vi "Magnetometer_Test_v1.vi"() -> ()   [LabVIEW 2019]
uses:
  <vilib>/DAQmx/write.llb/DAQmx Write (Analog DBL 1Chan 1Samp).vi
  <vilib>/DAQmx/read.llb/DAQmx Read (Analog 1D Wfm NChan NSamp).vi
  <extravilib>/ChannelInstances/Tag-bool/Write With Abort.vi
  <extravilib>/ChannelInstances/Tag-bool/Read With Abort.vi
  <extravilib>/ChannelInstances/Tag-c(bool,i32,str)/Read With Abort.vi
  <extravilib>/ChannelInstances/Tag-a[.](wfm(dbl))/Read With Abort.vi
  <extravilib>/ChannelInstances/Tag-c(bool,i32,str)/Write With Abort.vi
  <extravilib>/ChannelInstances/Tag-a[.](wfm(dbl))/Write With Abort.vi
  <vilib>/DAQmx/create/channels.llb/DAQmx Create Channel (AI-Voltage-Basic).vi
  <vilib>/DAQmx/configure/timing.llb/DAQmx Timing (Sample Clock).vi
  <vilib>/DAQmx/create/channels.llb/DAQmx Create Channel (AO-Voltage-Basic).vi
  <vilib>/Utility/file.llb/Write Delimited Spreadsheet (string).vi
  <extravilib>/ChannelInstances/Tag-a[.](wfm(dbl))/Instantiate.vi
  <extravilib>/ChannelInstances/Tag-bool/Instantiate.vi
  <extravilib>/ChannelInstances/Tag-bool/EndpointRead.vi
  <vilib>/DAQmx/miscellaneous.llb/DAQmx Fill In Error Info.vi
  <extravilib>/ChannelInstances/Tag-bool/Endpoint.vi
  <extravilib>/ChannelInstances/Tag-c(bool,i32,str)/Instantiate.vi
  <extravilib>/ChannelInstances/Tag-c(bool,i32,str)/EndpointRead.vi
  <extravilib>/ChannelInstances/Tag-a[.](wfm(dbl))/EndpointRead.vi
  <extravilib>/ChannelInstances/Tag-a[.](wfm(dbl))/Endpoint.vi
  <extravilib>/ChannelInstances/Tag-c(bool,i32,str)/Endpoint.vi
  <extravilib>/ChannelInstances/Tag-c(bool,i32,str).lvlib
  <extravilib>/ChannelInstances/Tag-a[.](wfm(dbl)).lvlib
  <extravilib>/ChannelInstances/Tag-bool.lvlib
  <resource>/objmgr/daqmx.rc
  <vilib>/DAQmx/write.llb/DAQmx Write (Analog 1D DBL NChan 1Samp).vi
panel:
  out "Temperature (VDC)":dbl
  out "Temperature":dbl(slide) scale=-40.0..160.0
  out "Magnetic Field Indicator":dbl
  out "Resistance (Ohms)":dbl
  out "Magnetic Field":dbl(graph)
  out "Temperature (Celsius)":dbl
  in  "MtM X-Axis Input Voltage":dbl
  in  "MtM Y-Axis Input Voltage":dbl
  in  "MtM Z-Axis Input Voltage":dbl
  in  "Simulation On/Off":bool
  in  "Temperature \nMeasurement On/Off":bool=TRUE
  in  "Data Record Work Rate (ms)":u16(ring)=100 items=["100"=100, "250"=250, "500"=500, "1000"=1000, "2500"=2500, "5000"=5000, ""=0]
  in  "Stop":bool
  out "Iteration of PS Controller":dbl
  out "Output 1 Measured Voltage":string
  out "Output 1 Input Voltage":string
  out "Output 1 Input Current":string
  out "Output 2 Measured Voltage":string
  out "Output 2 Measured Current":string
  out "Output 2 Input Voltage":string
  out "Output 1 Measured Current":string
  out "Output 2 Input Current":string
  in  "Reset":bool
  in  "Output On/Off":bool
  out "Output 1 Current In Range?":bool
  out "Output 2 Current In Range?":bool
  out "TCP Connection":bool
  out "MtM X-Axis Output Voltage":string
  in  "Data History Work Rate (ms)":u16(ring)=1000 items=["100"=100, "250"=250, "500"=500, "1000"=1000, "2500"=2500, "5000"=5000, ""=0]
  out "MtM Y-Axis Output Voltage":string
  out "MtM Z-Axis Output Voltage":string
  in  "Sample Clock Source":tag="OnboardClock"
  in  "Acquire Buffer Size":i32=1024
  out "While loop duration (ms)":u32
  out "DAQmx Read Rate":dbl
  in  "Number of Samples":i32=100
  out "MtM X-Axis Output Voltage 2":waveform(dbl)(graph)
  out "MtM Y-Axis Output Voltage 2":waveform(dbl)(graph)
  out "MtM Z-Axis Output Voltage 2":waveform(dbl)(graph)
  in  "Sample Rate":dbl=1000.0 format="%0.2f"
  # "Sensor Output"
  # "Data Acqusition Timing and\nBuffer Settings"
  # "Temperature Output"
  # "Acquire Data History"
  # "Magnetic Field Output"
  # "Power Supply Control and Status"
  # "Simulation of Analogue Voltage Generation"
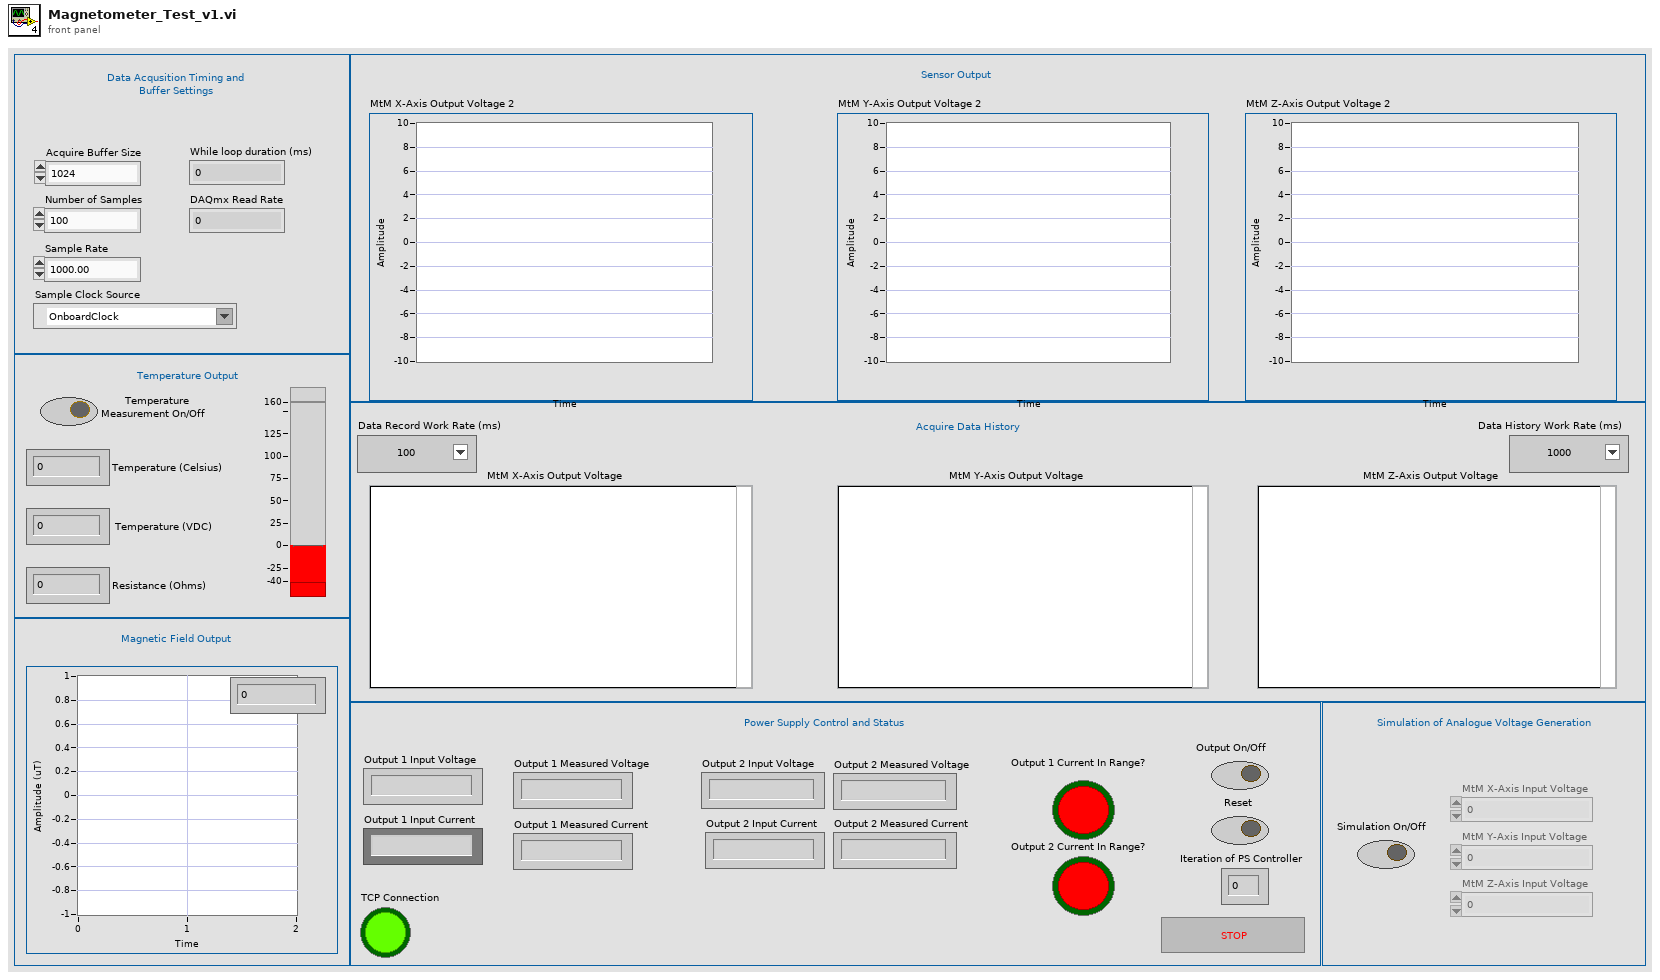
[diagram p1: front panel]
types:
  T1 = typedef "Tag-bool.lvlib/))Channel.ctl" = refnum<queue>
  T2 = enum8{"Enabled", "Disabled", "Disabled and Grayed Out"}
  T3 = typedef "Tag-a[.](wfm(dbl)).lvlib/))Channel.ctl" = refnum<queue>
  T4 = typedef "Tag-c(bool,i32,str).lvlib/))Channel.ctl" = refnum<queue>
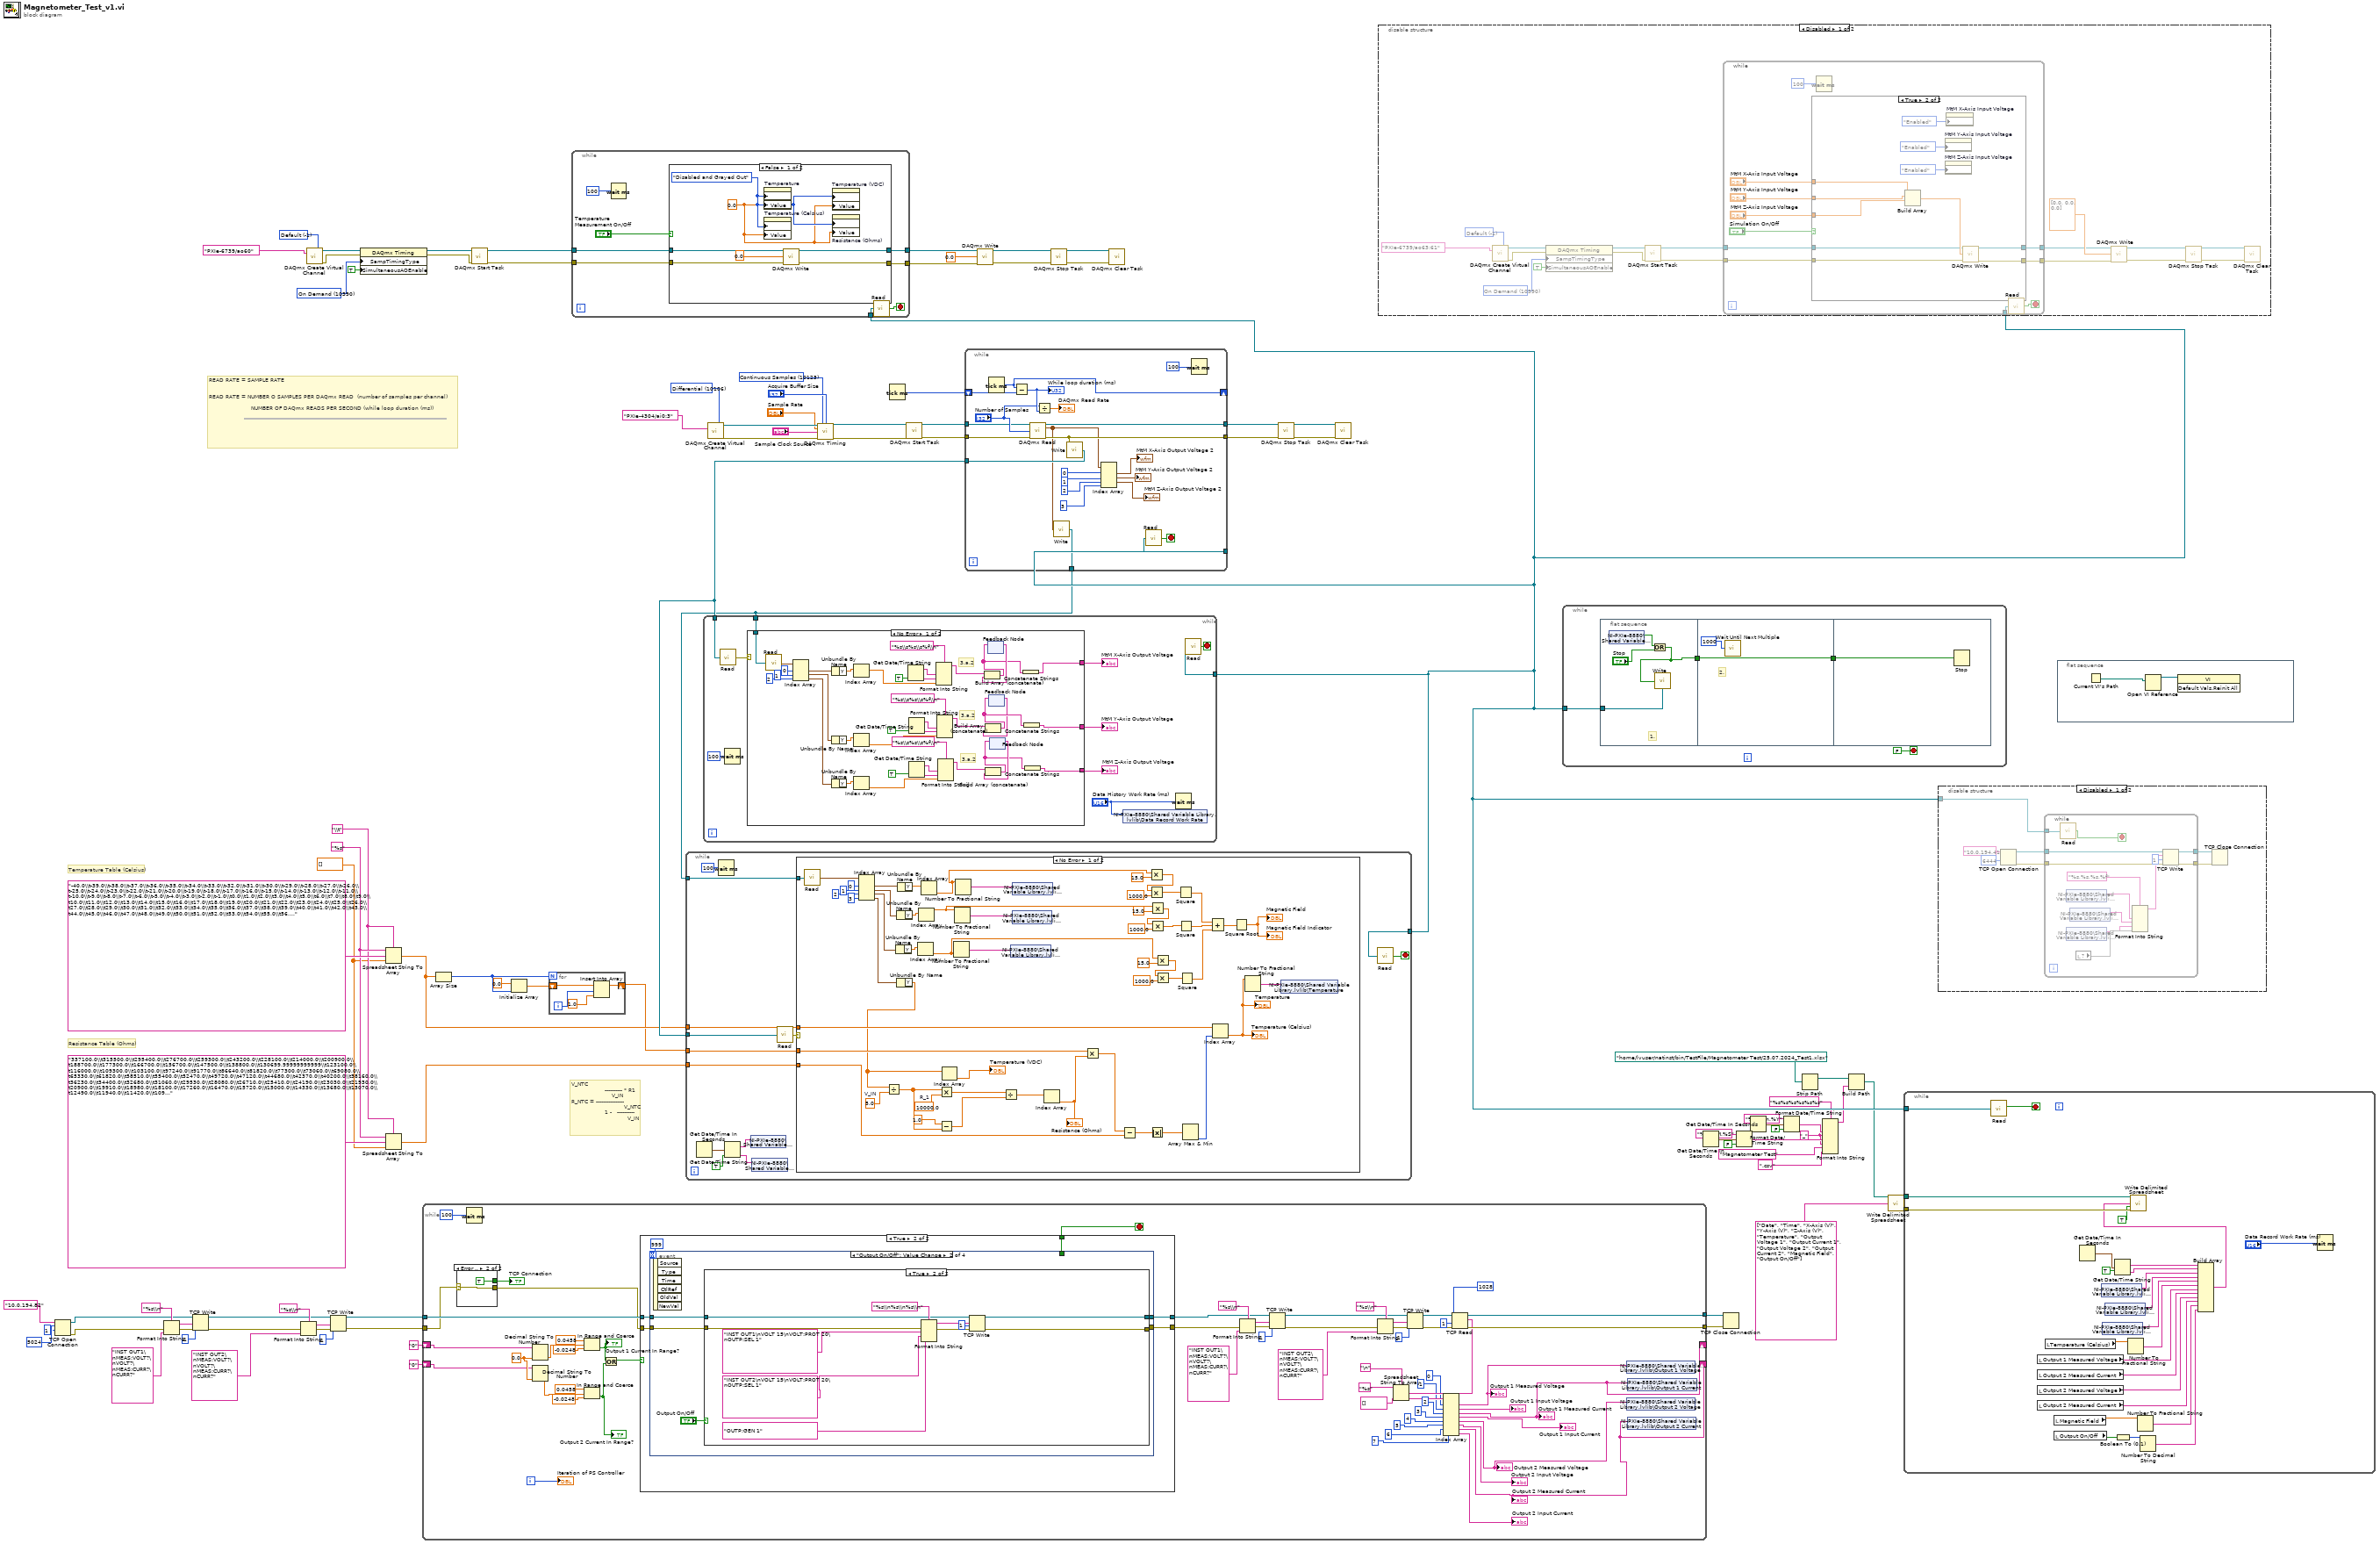
[diagram p0: block diagram]
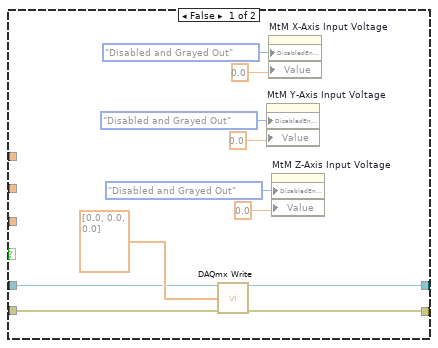
[diagram p4: hidden frame]
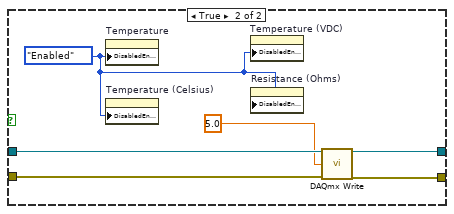
[diagram p6: hidden frame]
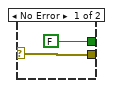
[diagram p7: hidden frame]
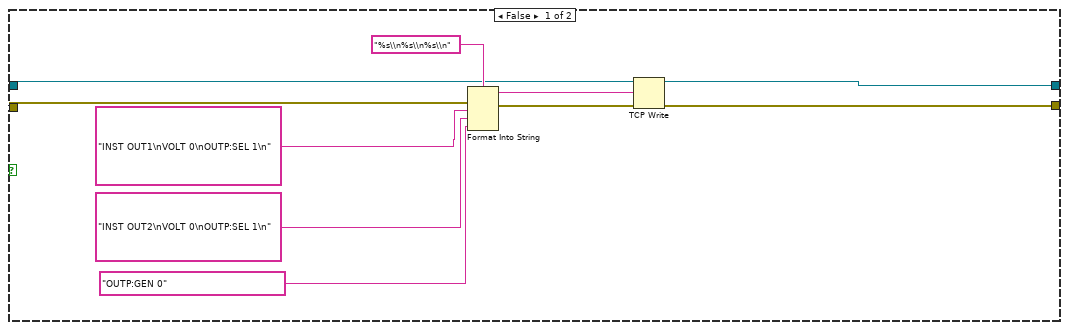
[diagram p8: hidden frame]
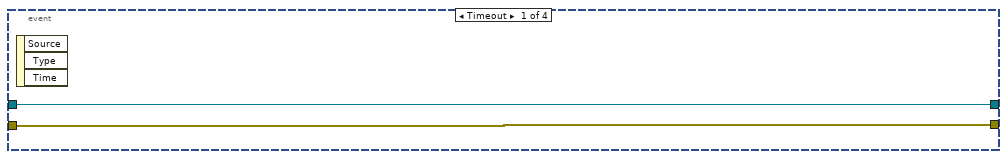
[diagram p9: hidden frame]
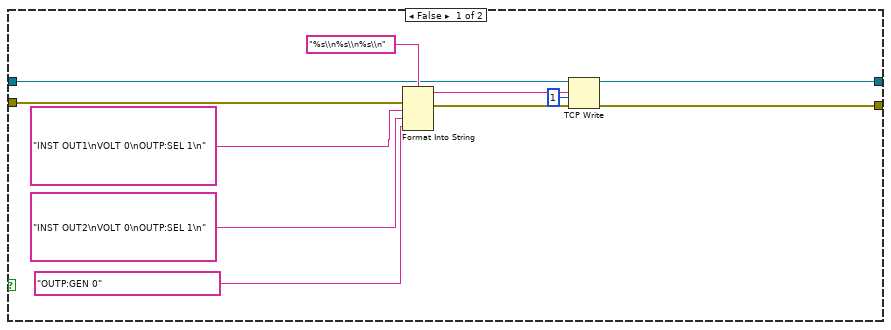
[diagram p10: hidden frame]
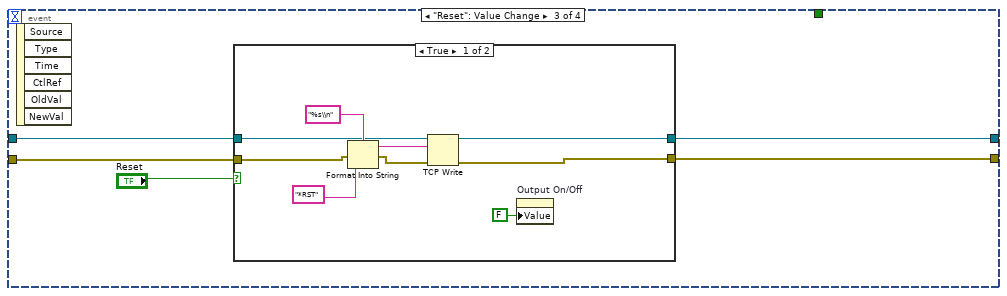
[diagram p11: hidden frame]
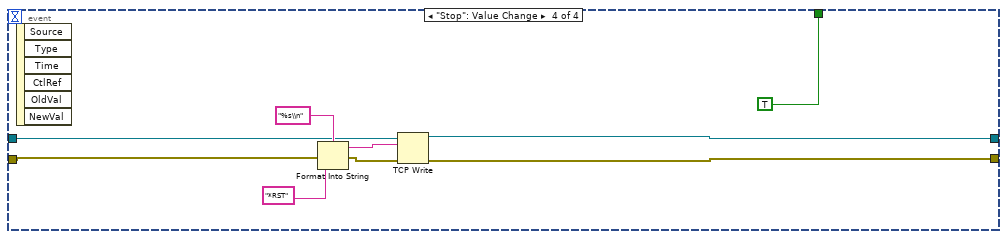
[diagram p13: hidden frame]
diagram:
  w12 = "\\t" ("delimiter (Tab)")
  w13 = "%s" ("format string")
  w8 = dbl[] [] ("array type (2D Dbl)")
  w16 = "_" ("input 2")
  w43 = 10390 items=["Sample Clock"=10388, "Burst Handshake"=12548, "Handshake"=10389, "Implicit"=10451, "On Demand"=10390, "Change Detection"=12504, "Pipelined Sample Clock"=14668] ("SampTimingType")
  w48 = -1 items=["Default"=-1, "RSE"=10083, "Differential"=10106, "Pseudodifferential"=12529] ("output terminal configuration")
  w77 = 10123 items=["Finite Samples"=10178, "Continuous Samples"=10123, "Hardware Timed Single Point"=12522] ("sample mode")
  w90 = 10106 items=["Default"=-1, "RSE"=10083, "NRSE"=10078, "Differential"=10106, "Pseudodifferential"=12529] ("input terminal configuration")
  # "V_NTC \n                   ---------- * R1 \n                       V_IN\nR_NTC = ----------------\n                              V_NTC \n                   1 -   ---------- \n                                V_IN"
  # "Resistance Table (Ohms)"
  # "Temperature Table (Celsius)"
  # "READ RATE = SAMPLE RATE\n\n\nREAD RATE = NUMBER O SAMPLES PER DAQmx READ  (number of samples per channel)\n\n                        NUMBER OF DAQmx READS PER SECOND (while loop duration (ms))"
  n1 = TCP Open Connection(address="10.0.194.82", remote port or service name=u16 5024, timeout ms (60000)=1) -> (connection ID=w51:refnum<k5>, error out=w52:errorcluster)  [unwired: 2 in]
  n2 = Format Into String(format string="%s\\n", error in=w52, "INST OUT1\nMEAS:VOLT?\nVOLT?\nMEAS:CURR?\nCURR?") -> (resulting string=w58:string, error out=w60:errorcluster)  [unwired: 1 in]
  n3 = TCP Write(connection ID=w51, data in=w58, error in (no error)=w60, 9:1 ("timeout ms (25000)")) -> (connection ID out=w56:refnum<k5>, error out=w55:errorcluster)  [unwired: 1 out]
  n4 = Format Into String(format string="%s\\n", error in=w55, "INST OUT2\nMEAS:VOLT?\nVOLT?\nMEAS:CURR?\nCURR?") -> (resulting string=w62:string, error out=w64:errorcluster)  [unwired: 1 in]
  n5 = call-poly <vilib>:"DAQmx Create Virtual Channel.vi"("output terminal configuration"=w48, "physical channels"=tag "PXIe-6739/ao60") -> ("task out"=w45:refnum<k21>, "error out"=w44:errorcluster)  [unwired: 12 in]
  n6 = TCP Write(connection ID=w56, data in=w62, error in (no error)=w64, 9:1 ("timeout ms (25000)")) -> (connection ID out=w54:refnum<k5>, error out=w53:errorcluster)  [unwired: 1 out]
  n7 = property class="DAQmx Timing"(reference=w45, error in=w44, "SampTimingType"=w43, "SimultaneousAOEnable"=TRUE) -> (reference out=w47:refnum<k21>, error out=w46:errorcluster)
  n8 = Spreadsheet String To Array(delimiter (Tab)=w12, format string=w13, spreadsheet string="-40,0\\t-39,0\\t-38,0\\t-37,0\\t-36,0\\t-35,0\\t-34,0\\t-33,0\\t-32,0\\t-31,0\\t-30,0\\t-29,0\\t-28,0\\t-27,0\\t-26,0\\t-25,0\\t-24,0\\t-23,0\\t-22,0\\t-21,0\\t-20,0\\t-19,0\\t-18,0\\t-17,0\\t-16,0\\t-15,0\\t-14,0\\t-13,0\\t-12,0\\t-11,0\\t-10,0\\t-9,0\\t-8,0\\t-7,0\\t-6,0\\t-5,0\\t-4,0\\t-3,0\\t-2,0\\t-1,0\\t0,0\\t1,0\\t2,0\\t3,0\\t4,0\\t5,0\\t6,0\\t7,0\\t8,0\\t9,0\\t10,0\\t11,0\\t12,0\\t13,0\\t14,0\\t15,0\\t16,0\\t17,0\\t18,0\\t19,0\\t20,0\\t21,0\\t22,0\\t23,0\\t24,0\\t25,0\\t26,0\\t27,0\\t28,0\\t29,0\\t30,0\\t31,0\\t32,0\\t33,0\\t34,0\\t35,0\\t36,0\\t37,0\\t38,0\\t39,0\\t40,0\\t41,0\\t42,0\\t43,0\\t44,0\\t45,0\\t46,0\\t47,0\\t48,0\\t49,0\\t50,0\\t51,0\\t52,0\\t53,0\\t54,0\\t55,0\\t56,0\\t57,0\\t58,0\\t59,0\\t60,0\\t61,0\\t62,0\\t63,0\\t64,0\\t65,0\\t66,0\\t67,0\\t68,0\\t69,0\\t70,0\\t71,0\\t72,0\\t73,0\\t74,0\\t75,0\\t76,0\\t77,0\\t78,0\\t79,0\\t80,0\\t81,0\\t82,0\\t83,0\\t84,0\\t85,0\\t86,0\\t87,0\\t88,0\\t89,0\\t90,0\\t91,0\\t92,0\\t93,0\\t94,0\\t95,0\\t96,0\\t97,0\\t98,0\\t99,0\\t100,0\\t101,0\\t102,0\\t103,0\\t104,0\\t105,0\\t106,0\\t107,0\\t108,0\\t109,0\\t110,0\\t111,0\\t112,0\\t113,0\\t114,0\\t115,0\\t116,0\\t117,0\\t118,0\\t119,0\\t120,0\\t121,0\\t122,0\\t123,0\\t124,0\\t125,0\\t126,0\\t127,0\\t128,0\\t129,0\\t130,0\\t131,0\\t132,0\\t133,0\\t134,0\\t135,0\\t136,0\\t137,0\\t138,0\\t139,0\\t140,0\\t141,0\\t142,0\\t143,0\\t144,0\\t145,0\\t146,0\\t147,0\\t148,0\\t149,0\\t150,0\\t151,0\\t152,0\\t153,0\\t154,0\\t155,0\\t156,0\\t157,0\\t158,0\\t159,0\\t160,0\\t161,0\\t162,0\\t163,0\\t164,0\\t165,0\\t166,0\\t167,0\\t168,0\\t169,0\\t170,0\\t171,0\\t172,0\\t173,0\\t174,0\\t175,0\\t176,0\\t177,0\\t178,0\\t179,0\\t180,0\\t181,0\\t182,0\\t183,0\\t184,0\\t185,0\\t186,0\\t187,0\\t188,0\\t189,0\\t190,0\\t191,0\\t192,0\\t193,0\\t194,0\\t195,0\\t196,0\\t197,0\\t198,0\\t199,0\\t200,0\\t201,0\\t202,0\\t203,0\\t204,0\\t205,0\\t206,0\\t207,0\\t208,0\\t209,0\\t210,0\\t211,0\\t212,0\\t213,0\\t214,0\\t215,0\\t216,0\\t217,0\\t218,0\\t219,0\\t220,0\\t221,0\\t222,0\\t223,0\\t224,0\\t225,0\\t226,0\\t227,0\\t228,0\\t229,0\\t230,0\\t231,0\\t232,0\\t233,0\\t234,0\\t235,0\\t236,0\\t237,0\\t238,0\\t239,0\\t240,0\\t241,0\\t242,0\\t243,0\\t244,0\\t245,0\\t246,0\\t247,0\\t248,0\\t249,0\\t250,0", array type (2D Dbl)=w8) -> (array=w10:dbl[])
  n9 = Spreadsheet String To Array(delimiter (Tab)=w12, format string=w13, spreadsheet string="337100,0\\t315500,0\\t295400,0\\t276700,0\\t259300,0\\t243200,0\\t228100,0\\t214000,0\\t200900,0\\t188700,0\\t177300,0\\t166700,0\\t156700,0\\t147500,0\\t138800,0\\t130699,99999999999\\t123100,0\\t116000,0\\t109300,0\\t103100,0\\t97240,0\\t91770,0\\t86640,0\\t81820,0\\t77300,0\\t73060,0\\t69080,0\\t65330,0\\t61820,0\\t58510,0\\t55400,0\\t52470,0\\t49720,0\\t47120,0\\t44680,0\\t42370,0\\t40200,0\\t38160,0\\t36230,0\\t34400,0\\t32680,0\\t31060,0\\t29530,0\\t28080,0\\t26710,0\\t25410,0\\t24190,0\\t23030,0\\t21930,0\\t20900,0\\t19910,0\\t18980,0\\t18100,0\\t17260,0\\t16470,0\\t15720,0\\t15000,0\\t14330,0\\t13680,0\\t13070,0\\t12490,0\\t11940,0\\t11420,0\\t10920,0\\t10450,0\\t10000,0\\t9572,0\\t9164,0\\t8776,0\\t8407,0\\t8055,0\\t7720,0\\t7401,0\\t7097,0\\t6806,0\\t6530,0\\t6266,0\\t6014,0\\t5773,0\\t5544,0\\t5325,0\\t5115,0\\t4915,0\\t4724,0\\t4542,0\\t4367,0\\t4200,0\\t4041,0000000000005\\t3888,0\\t3742,0\\t3602,0\\t3468,0\\t3339,0\\t3217,0\\t3099,0\\t2986,0\\t2878,0\\t2774,0\\t2675,0\\t2580,0\\t2488,0\\t2401,0\\t2317,0\\t2236,0\\t2158,0\\t2084,0\\t2012,0\\t1944,0\\t1878,0\\t1814,0\\t1753,0\\t1695,0\\t1639,0\\t1584,0\\t1532,0\\t1482,0\\t1434,0\\t1387,0\\t1343,0\\t1300,0\\t1258,0\\t1218,0\\t1180,0\\t1143,0\\t1107,0\\t1073,0\\t1039,0\\t1006,9999999999999\\t976,6\\t946,8\\t918,1\\t890,4\\t863,7\\t837,9\\t813,0\\t789,0\\t765,8000000000001\\t743,4\\t721,7\\t700,8\\t680,6\\t661,0\\t642,1\\t623,9\\t606,1999999999999\\t589,1999999999999\\t572,6999999999999\\t556,6999999999999\\t541,3\\t526,3\\t511,90000000000003\\t497,90000000000003\\t484,3\\t471,2\\t458,5\\t446,2\\t434,3\\t422,70000000000005\\t411,5\\t400,7\\t390,2\\t380,0\\t370,2\\t360,59999999999997\\t351,3\\t342,3\\t333,6\\t325,2\\t316,90000000000003\\t309,0\\t301,3\\t293,8\\t286,5\\t279,4\\t272,5\\t265,90000000000003\\t259,40000000000003\\t253,1\\t247,0\\t241,10000000000002\\t235,3\\t229,7\\t224,3\\t219,0\\t213,9\\t208,9\\t204,0\\t199,3\\t194,70000000000002\\t190,20000000000002\\t185,9\\t181,7\\t177,5\\t173,5\\t169,6\\t165,8\\t162,20000000000002\\t158,6\\t155,1\\t151,7\\t148,29999999999998\\t145,1\\t142,0\\t138,9\\t135,9\\t133,0\\t130,20000000000002\\t127,40000000000002\\t124,7\\t122,1\\t119,5\\t117,0\\t114,6\\t112,19999999999999\\t109,89999999999999\\t107,7\\t105,5\\t103,3\\t101,2\\t99,2\\t97,19999999999999\\t95,2\\t93,3\\t91,5\\t89,7\\t87,9\\t86,2\\t84,5\\t82,9\\t81,3\\t79,69999999999999\\t78,2\\t76,7\\t75,2\\t73,80000000000001\\t72,4\\t71,0\\t69,7\\t68,4\\t67,10000000000001\\t65,9\\t64,69999999999999\\t63,5\\t62,300000000000004\\t61,199999999999996\\t60,1\\t59,0\\t57,9\\t56,9\\t55,9\\t54,9\\t53,900000000000006\\t53,0\\t52,0\\t51,1\\t50,2\\t49,4\\t48,5\\t47,7\\t46,800000000000004\\t46,0\\t45,3\\t44,5\\t43,7\\t43,0\\t42,3\\t41,6\\t40,9\\t40,2\\t39,5\\t38,9\\t38,199999999999996\\t37,6\\t37,0\\t36,4\\t35,8\\t35,2\\t34,7\\t34,1\\t33,6\\t33,0\\t32,5\\t32,0\\t31,5\\t31,0\\t30,5\\t30,099999999999998\\t29,6\\t29,1\\t28,7\\t28,299999999999997", array type (2D Dbl)=w8) -> (array=w7:dbl[])
  n10 = while {
    tunnel: w54 -> [w147]
    tunnel: w53 -> [w97]
    tunnel: [w150] -> w71
    tunnel: [w149] -> w70
    shift-right: [w94] -> _
    shift-left: "0" -> [w93]
    shift-right: [w92] -> _
    shift-left: "0" -> [w91]
    i -> [w148]
    stop <- w146 stop-if-true
    w145 = 0.0
    n11 = case shown="Error .." w97 {
      selector: w97 -> [w151 w153]
      tunnel: [FALSE ("TCP Connection") TRUE ("TCP Connection")] -> w96
      tunnel: [w151 w153] -> w95
      frame No Error {
      }
      frame Error {
      }
    }
    "TCP Connection" <- w96
    n12 = Wait (ms)(milliseconds to wait=u32 100 ("millisecond multiple")) -> ()  [unwired: 1 out]
    n13 = Decimal String To Number(string=w93, default (0L)=w145) -> (number=w139:dbl)  [unwired: 1 in, 1 out]
    n14 = Decimal String To Number(string=w91, default (0L)=w145) -> (number=w138:dbl)  [unwired: 1 in, 1 out]
    n15 = In Range and Coerce(upper limit=0.0458 ("y"), x=w138, lower limit=-0.0248 ("y")) -> (In Range?=w124:bool)  [unwired: 1 out]
    "Output 2 Current In Range?" <- w124
    n16 = In Range and Coerce(upper limit=0.0458 ("y"), x=w139, lower limit=-0.0248 ("y")) -> (In Range?=w137:bool)  [unwired: 1 out]
    "Output 1 Current In Range?" <- w137
    n17 = Or(x=w137, y=w124) -> (x .or. y?=w125:bool)
    n18 = case shown="True" w125 {
      tunnel: w147 -> [w158 w170]
      tunnel: w95 -> [w157 w169]
      tunnel: [_ w168] -> w146
      tunnel: [w155 w166] -> w100
      tunnel: [w156 w165] -> w99
      frame False {
        n19 = Format Into String(format string="%s\\n%s\\n%s\\n", error in=w157, "INST OUT1\nVOLT 0\nOUTP:SEL 1\n", "INST OUT2\nVOLT 0\nOUTP:SEL 1\n", "OUTP:GEN 0") -> (resulting string=w163:string, error out=w164:errorcluster)  [unwired: 1 in]
        n20 = TCP Write(connection ID=w158, data in=w163, error in (no error)=w164) -> (connection ID out=w155:refnum<k5>, error out=w156:errorcluster)  [unwired: 1 in, 1 out]
      }
      frame True {
        n21 = event shown="[1] \"Output On/Off\": Value Change" {
          selector: _ -> [_ _ _ _]
          dyn-events: _ -> [_ _ _ _]
          timeout: 999 -> [_ _ _ _]
          tunnel: [w171 w177 w202 w217] -> w166
          tunnel: [w172 w175 w201 w216] -> w165
          tunnel: w170 -> [w171 w174 w204 w219]
          tunnel: w169 -> [w172 w173 w203 w220]
          tunnel: [_ _ _ TRUE] -> w168
          event Timeout {
            n22 = event-data() -> ()  [unwired: 1 in, 3 out]
          }
          event "Output On/Off": Value Change {
            n23 = event-data() -> ()  [unwired: 1 in, 6 out]
            n24 = case shown="True" "Output On/Off" {
              tunnel: [w180 w194] -> w177
              tunnel: [w179 w193] -> w175
              tunnel: w174 -> [w182 w196]
              tunnel: w173 -> [w181 w195]
              frame False {
                n25 = Format Into String(format string="%s\\n%s\\n%s\\n", error in=w181, "INST OUT1\nVOLT 0\nOUTP:SEL 1\n", "INST OUT2\nVOLT 0\nOUTP:SEL 1\n", "OUTP:GEN 0") -> (resulting string=w187:string, error out=w188:errorcluster)  [unwired: 1 in]
                n26 = TCP Write(connection ID=w182, data in=w187, error in (no error)=w188, 9:1 ("timeout ms (25000)")) -> (connection ID out=w180:refnum<k5>, error out=w179:errorcluster)  [unwired: 1 out]
              }
              frame True {
                n27 = Format Into String(format string="%s\\n%s\\n%s\\n", error in=w195, "INST OUT1\nVOLT 15\nVOLT:PROT 20\nOUTP:SEL 1", "INST OUT2\nVOLT 15\nVOLT:PROT 20\nOUTP:SEL 1", "OUTP:GEN 1") -> (resulting string=w197:string, error out=w199:errorcluster)  [unwired: 1 in]
                n28 = TCP Write(connection ID=w196, data in=w197, error in (no error)=w199, 9:1 ("timeout ms (25000)")) -> (connection ID out=w194:refnum<k5>, error out=w193:errorcluster)  [unwired: 1 out]
              }
            }
          }
          event "Reset": Value Change {
            n29 = event-data() -> ()  [unwired: 1 in, 6 out]
            n30 = case shown="True" "Reset" {
              tunnel: [w207 w215] -> w202
              tunnel: [w206 w214] -> w201
              tunnel: w204 -> [w208 w215]
              tunnel: w203 -> [w209 w214]
              frame True {
                n31 = Format Into String(format string="%s\\n", error in=w209, "*RST" ("data in")) -> (resulting string=w211:string, error out=w210:errorcluster)  [unwired: 1 in]
                n32 = TCP Write(connection ID=w208, data in=w211, error in (no error)=w210) -> (connection ID out=w207:refnum<k5>, error out=w206:errorcluster)  [unwired: 1 in, 1 out]
                n33 = property on="Output On/Off" class="Bool (strict)"("Value"=FALSE ("Output On/Off")) -> ()  [unwired: 2 in, 2 out]
              }
              frame False {
              }
            }
          }
          event "Stop": Value Change {
            n34 = event-data() -> ()  [unwired: 1 in, 6 out]
            n35 = Format Into String(format string="%s\\n", error in=w220, "*RST" ("data in")) -> (resulting string=w222:string, error out=w221:errorcluster)  [unwired: 1 in]
            n36 = TCP Write(connection ID=w219, data in=w222, error in (no error)=w221) -> (connection ID out=w217:refnum<k5>, error out=w216:errorcluster)  [unwired: 1 in, 1 out]
          }
        }
      }
    }
    n37 = Format Into String(format string="%s\\n", error in=w99, "INST OUT1\nMEAS:VOLT?\nVOLT?\nMEAS:CURR?\nCURR?") -> (resulting string=w104:string, error out=w106:errorcluster)  [unwired: 1 in]
    n38 = TCP Write(connection ID=w100, data in=w104, error in (no error)=w106, 9:1 ("timeout ms (25000)")) -> (connection ID out=w102:refnum<k5>, error out=w101:errorcluster)  [unwired: 1 out]
    n39 = Format Into String(format string="%s\\n", error in=w101, "INST OUT2\nMEAS:VOLT?\nVOLT?\nMEAS:CURR?\nCURR?") -> (resulting string=w129:string, error out=w131:errorcluster)  [unwired: 1 in]
    n40 = TCP Write(connection ID=w102, data in=w129, error in (no error)=w131, 9:1 ("timeout ms (25000)")) -> (connection ID out=w128:refnum<k5>, error out=w127:errorcluster)  [unwired: 1 out]
    n41 = TCP Read(connection ID=w128, bytes to read=1028, error in (no error)=w127, 9:1 ("timeout ms (25000)")) -> (connection ID out=w150:refnum<k5>, data out=w132:string, error out=w149:errorcluster)  [unwired: 1 in]
    n42 = Spreadsheet String To Array(delimiter (Tab)="\n", format string="%s", spreadsheet string=w132, array type (2D Dbl)=string[] []) -> (array=w134:string[])
    n43 = Index Array(array=w134, index #1=0 ("index"), index #2=1 ("index"), index #3=2 ("index"), index #4=3 ("index"), index #5=4 ("index"), index #6=5 ("index"), index #7=6 ("index"), index #8=7 ("index")) -> (element #1=w123:string, element #2=→"Output 1 Input Voltage":string, element #3=w94:string, element #4=→"Output 1 Input Current":string, element #5=w119:string, element #6=→"Output 2 Input Voltage":string, element #7=w92:string, element #8=→"Output 2 Input Current":string)
    "Output 1 Measured Voltage" <- w123
    "Output 2 Measured Voltage" <- w119
    "Output 2 Measured Current" <- w92
    "Output 1 Measured Current" <- w94
    n44 = shared-variable "NI-PXIe-8880\\Shared Variable Library.lvlib\\Output 1 Voltage"(w123) -> ()  [unwired: 1 in, 1 out]
    n45 = shared-variable "NI-PXIe-8880\\Shared Variable Library.lvlib\\Output 2 Voltage"(w119) -> ()  [unwired: 1 in, 1 out]
    n46 = shared-variable "NI-PXIe-8880\\Shared Variable Library.lvlib\\Output 2 Current"(w92) -> ()  [unwired: 1 in, 1 out]
    n47 = shared-variable "NI-PXIe-8880\\Shared Variable Library.lvlib\\Output 1 Current"(w94) -> ()  [unwired: 1 in, 1 out]
    "Iteration of PS Controller" <- w148
  }
  n48 = Array Size(array=w10) -> (size(s)=w11:i32)
  n49 = call <vilib>:"DAQmx Start Task.vi"("task/channels in"=w47, "error in"=w46) -> ("task out"=w40:refnum<k21>, "error out"=w39:errorcluster)  [unwired: 12 in]
  n50 = Initialize Array(0.0 ("element"), w11) -> (w4:dbl[])
  n51 = for {
    N: w11 -> [_]
    shift-right: [w227] -> w9
    shift-left: w4 -> [w228]
    i -> [w226]
    n52 = Insert Into Array(array=w228, index=w226, new element=1.0 ("new element/subarray")) -> (w227:dbl[])
  }
  n53 = call-poly <vilib>:"DAQmx Create Virtual Channel.vi"("input terminal configuration"=w90, "physical channels"=tag "PXIe-4304/ai0:3") -> ("task out"=w82:refnum<k21>, "error out"=w81:errorcluster)  [unwired: 12 in]
  n54 = call-poly <vilib>:"DAQmx Timing.vi"("task/channels in"=w82, "sample mode"=w77, "samples per channel"="Acquire Buffer Size", "rate"="Sample Rate", "source"="Sample Clock Source", "error in"=w81) -> ("task out"=w79:refnum<k21>, "error out"=w80:errorcluster)  [unwired: 8 in]
  n55 = Tick Count (ms)() -> (millisecond timer value=w83:u32)
  n56 = call <vilib>:"DAQmx Start Task.vi"("task/channels in"=w79, "error in"=w80) -> ("task out"=w88:refnum<k21>, "error out"=w89:errorcluster)  [unwired: 12 in]
  n57 = while {
    tunnel: [w230] -> w28
    stop <- FALSE stop-if-true
    n58 = flat-sequence {
      tunnel: [w233] -> w231
      tunnel: [w236] -> w230
      tunnel: w231 -> [w238]
      tunnel: [w238] -> w229
      tunnel: w229 -> [w239]
      frame #0 {
        # "1."
        n59 = shared-variable "NI-PXIe-8880\\Shared Variable Library.lvlib\\Stop"() -> (w234:bool)  [unwired: 1 in, 1 out]
        n60 = Or(x=w234, y="Stop") -> (x .or. y?=w233:bool)
        n61 = call <extravilib>:"Write.vi"("element"=w233) -> ("channel"=w236:T1)  [unwired: 1 out]
      }
      frame #1 {
        # "2."
        n62 = call "Wait Until Next Multiple"("Count(mSec)"=u32 1000) -> ()  [unwired: 1 out]
      }
      frame #2 {
        n63 = Stop(stop? (T)=w239) -> ()
      }
    }
  }
  n64 = while {
    tunnel: w40 -> [w247]
    tunnel: w39 -> [w246]
    tunnel: [w245] -> w34
    tunnel: [w244] -> w33
    tunnel: w28 -> [w243]
    stop <- w242 stop-if-true
    n65 = Wait (ms)(milliseconds to wait=u32 100) -> ()  [unwired: 1 out]
    n66 = case shown="False" "Temperature \nMeasurement On/Off" {
      tunnel: w247 -> [w252 w260]
      tunnel: w246 -> [w251 w259]
      tunnel: [w254 w258] -> w245
      tunnel: [w253 w257] -> w244
      frame False {
        w248 = 0.0 ("Temperature")
        w249 = T2."Disabled and Grayed Out" ("Disabled")
        n67 = property on="Temperature" class="Slide (strict)"("DisabledEnum"=w249, "Value"=w248) -> ()  [unwired: 2 in, 2 out]
        n68 = property on="Temperature (Celsius)" class="DigNum (strict)"("DisabledEnum"=w249, "Value"=w248) -> ()  [unwired: 2 in, 2 out]
        n69 = call-poly <vilib>:"DAQmx Write.vi"("task/channels in"=w252, "data"=0.0 ("Waveform"), "error in"=w251) -> ("task out"=w254:refnum<k21>, "error out"=w253:errorcluster)  [unwired: 10 in, 1 out]
        n70 = property on="Temperature (VDC)" class="DigNum (strict)"("DisabledEnum"=w249, "Value"=w248) -> ()  [unwired: 2 in, 2 out]
        n71 = property on="Resistance (Ohms)" class="DigNum (strict)"("DisabledEnum"=w249, "Value"=w248) -> ()  [unwired: 2 in, 2 out]
      }
      frame True {
        w255 = T2."Enabled" ("Disabled")
        n72 = property on="Temperature" class="Slide (strict)"("DisabledEnum"=w255) -> ()  [unwired: 2 in, 2 out]
        n73 = property on="Temperature (Celsius)" class="DigNum (strict)"("DisabledEnum"=w255) -> ()  [unwired: 2 in, 2 out]
        n74 = property on="Temperature (VDC)" class="DigNum (strict)"("DisabledEnum"=w255) -> ()  [unwired: 2 in, 2 out]
        n75 = property on="Resistance (Ohms)" class="DigNum (strict)"("DisabledEnum"=w255) -> ()  [unwired: 2 in, 2 out]
        n76 = call-poly <vilib>:"DAQmx Write.vi"("task/channels in"=w260, "data"=5.0 ("MtM X-Axis Input Voltage 2"), "error in"=w259) -> ("task out"=w258:refnum<k21>, "error out"=w257:errorcluster)  [unwired: 10 in, 1 out]
      }
    }
    n77 = call <extravilib>:"Read.vi"("channel"=w243) -> ("element"=w242:bool)  [unwired: 1 in, 1 out]
  }
  n78 = while {
    shift-right: [w277] -> _
    shift-left: w83 -> [w280]
    tunnel: w88 -> [w274]
    tunnel: [w282] -> w87
    tunnel: w89 -> [w273]
    tunnel: [w281] -> w86
    tunnel: [w267] -> w31
    tunnel: [w265] -> w5
    tunnel: w28 -> [w264]
    stop <- w263 stop-if-true
    n79 = Tick Count (ms)() -> (millisecond timer value=w277:u32)
    n80 = Subtract(x=w277, y=w280) -> (x-y=w276:u32)
    "While loop duration (ms)" <- w276
    n81 = call-poly <vilib>:"DAQmx Read.vi"("task/channels in"=w274, "number of samples per channel"="Number of Samples", "error in"=w273) -> ("task out"=w282:refnum<k21>, "data"=w266:waveform(dbl)[], "error out"=w281:errorcluster)  [unwired: 10 in]
    n82 = Divide(x="Number of Samples", y=w276) -> (x/y=→"DAQmx Read Rate":dbl)
    n83 = call <extravilib>:"Write.vi"("element"=w266) -> ("channel"=w265:T3)  [unwired: 1 out]
    n84 = call <extravilib>:"Write.vi"("element"=w281) -> ("channel"=w267:T4)  [unwired: 1 out]
    n85 = Index Array(array=w266, index #1=0 ("index"), index #2=1 ("index"), index #3=2 ("index"), index #4=3 ("index")) -> (element #1=→"MtM X-Axis Output Voltage 2":waveform(dbl), element #2=→"MtM Y-Axis Output Voltage 2":waveform(dbl), element #3=→"MtM Z-Axis Output Voltage 2":waveform(dbl))  [unwired: 1 out]
    n86 = call <extravilib>:"Read.vi"("channel"=w264) -> ("element"=w263:bool)  [unwired: 1 in, 1 out]
    n87 = Wait (ms)(milliseconds to wait=u32 100) -> ()  [unwired: 1 out]
  }
  n88 = while {
    tunnel: w28 -> [w294]
    tunnel: w31 -> [w292]
    tunnel: w7 -> [w285]
    tunnel: w10 -> [w284]
    tunnel: w9 -> [w286]
    tunnel: w5 -> [w283]
    stop <- w295 stop-if-true
    n89 = Get Date/Time In Seconds() -> (seconds since 1Jan1904=w289:timestamp)
    n90 = Wait (ms)(milliseconds to wait=u32 100) -> ()  [unwired: 1 out]
    n91 = Get Date/Time String(seconds (now)=w289, want seconds? (F)=TRUE) -> (date string=w290:string, time string=w291:string)  [unwired: 1 in]
    n92 = shared-variable "NI-PXIe-8880\\Shared Variable Library.lvlib\\Date"(w290) -> ()  [unwired: 1 in, 1 out]
    n93 = shared-variable "NI-PXIe-8880\\Shared Variable Library.lvlib\\Time"(w291) -> ()  [unwired: 1 in, 1 out]
    n94 = call <extravilib>:"Read.vi"("channel"=w292) -> ("element"=w293:errorcluster)  [unwired: 1 in, 1 out]
    n95 = case shown="No Error" w293 {
      tunnel: w283 -> [w326 _]
      tunnel: w284 -> [w304 _]
      tunnel: w286 -> [w306 _]
      tunnel: w285 -> [w310 _]
      frame No Error {
        w315 = 10000.0  # R_1
        w316 = 5.0  # V_IN
        n96 = call <extravilib>:"Read.vi"("channel"=w326) -> ("element"=w325:waveform(dbl)[])  [unwired: 1 in, 1 out]
        n97 = Index Array(array=w325, index #1=0 ("index"), index #2=1 ("index"), index #3=2 ("index"), index #4=3 ("index")) -> (element #1=w324:waveform(dbl), element #2=w323:waveform(dbl), element #3=w319:waveform(dbl), element #4=w321:waveform(dbl))
        n98 = Unbundle By Name(w319) -> ("Y"=w320:dbl[])
        n99 = Unbundle By Name(w323) -> ("Y"=w322:dbl[])
        n100 = Unbundle By Name(w321) -> ("Y"=w303:dbl[])
        n101 = Divide(x=w303, y=w316) -> (x/y=w312:dbl[])
        n102 = Unbundle By Name(w324) -> ("Y"=w318:dbl[])
        n103 = Index Array(array=w320) -> (element=w327:dbl)  [unwired: 1 in]
        n104 = Index Array(array=w322) -> (element=w328:dbl)  [unwired: 1 in]
        n105 = Index Array(array=w318) -> (element=w317:dbl)  [unwired: 1 in]
        n106 = Multiply(x=w312, y=w315) -> (x*y=w314:dbl[])
        n107 = Subtract(x=1.0, y=w312) -> (x-y=w311:dbl[])
        n108 = Index Array(array=w303) -> (element=→"Temperature (VDC)":dbl)  [unwired: 1 in]
        n109 = Number To Fractional String(number=w327) -> (F-format string=w344:string)  [unwired: 3 in]
        n110 = Number To Fractional String(number=w328) -> (F-format string=w345:string)  [unwired: 3 in]
        n111 = Number To Fractional String(number=w317) -> (F-format string=w346:string)  [unwired: 3 in]
        n112 = Divide(x=w314, y=w311) -> (x/y=w300:dbl[])
        n113 = shared-variable "NI-PXIe-8880\\Shared Variable Library.lvlib\\Z-Axis"(w344) -> ()  [unwired: 1 in, 1 out]
        n114 = shared-variable "NI-PXIe-8880\\Shared Variable Library.lvlib\\Y-Axis"(w345) -> ()  [unwired: 1 in, 1 out]
        n115 = shared-variable "NI-PXIe-8880\\Shared Variable Library.lvlib\\X-Axis"(w346) -> ()  [unwired: 1 in, 1 out]
        n116 = Index Array(array=w300) -> (element=w301:dbl)  [unwired: 1 in]
        "Resistance (Ohms)" <- w301
        n117 = Multiply(x=w306, y=w301) -> (x*y=w307:dbl[])
        n118 = Subtract(x=w307, y=w310) -> (x-y=w305:dbl[])
        n119 = Multiply(x=w317, y=15.0) -> (x*y=w342:dbl)
        n120 = Multiply(x=w342, y=1000.0) -> (x*y=w338:dbl)
        n121 = Absolute Value(x=w305) -> (abs(x)=w309:dbl[])
        n122 = Multiply(x=w328, y=15.0) -> (x*y=w337:dbl)
        n123 = Multiply(x=w337, y=1000.0) -> (x*y=w336:dbl)
        n124 = Multiply(x=w327, y=15.0) -> (x*y=w332:dbl)
        n125 = Multiply(x=w332, y=1000.0) -> (x*y=w333:dbl)
        n126 = Square(x=w338) -> (x^2=w330:dbl)
        n127 = Square(x=w336) -> (x^2=w331:dbl)
        n128 = Square(x=w333) -> (x^2=w329:dbl)
        n129 = Array Max & Min(array=w309) -> (min index (indices)=w308:i32)  [unwired: 3 out]
        n130 = Compound Arithmetic op=ADD(w330, w331, w329) -> (w299:dbl)
        n131 = Index Array "Index Array"(array=w304, index=w308) -> (element=w297:dbl)
        "Temperature (Celsius)" <- w297
        "Temperature" <- w297
        n132 = Square Root(x=w299) -> (sqrt(x)=→"Magnetic Field" →"Magnetic Field Indicator":dbl)
        n133 = Number To Fractional String(number=w297) -> (F-format string=w296:string)  [unwired: 3 in]
        n134 = shared-variable "NI-PXIe-8880\\Shared Variable Library.lvlib\\Temperature"(w296) -> ()  [unwired: 1 in, 1 out]
      }
      frame Error {
      }
    }
    n135 = call <extravilib>:"Read.vi"("channel"=w294) -> ("element"=w295:bool)  [unwired: 1 in, 1 out]
  }
  n136 = while {
    tunnel: w31 -> [w360]
    tunnel: w5 -> [w359]
    tunnel: w28 -> [w358]
    stop <- w357 stop-if-true
    n137 = call <extravilib>:"Read.vi"("channel"=w360) -> ("element"=w356:errorcluster)  [unwired: 1 in, 1 out]
    n138 = Wait (ms)(milliseconds to wait=u32 100) -> ()  [unwired: 1 out]
    n139 = case shown="No Error" w356 {
      tunnel: w359 -> [w393 _]
      tunnel: [w386 _] -> w355
      tunnel: [w378 _] -> w354
      tunnel: [w377 _] -> w353
      frame No Error {
        # "3.a.2"
        # "3.a.2"
        # "3.a.2"
        n140 = call <extravilib>:"Read.vi"("channel"=w393) -> ("element"=w389:waveform(dbl)[])  [unwired: 1 in, 1 out]
        n141 = Index Array(array=w389, index #1=0 ("index"), index #2=1 ("index"), index #3=2 ("index")) -> (element #1=w369:waveform(dbl), element #2=w368:waveform(dbl), element #3=w367:waveform(dbl))
        n142 = Unbundle By Name(w369) -> ("Y"=w366:dbl[])
        n143 = Unbundle By Name(w368) -> ("Y"=w365:dbl[])
        n144 = Unbundle By Name(w367) -> ("Y"=w364:dbl[])
        n145 = Index Array(array=w366) -> (element=w361:dbl)  [unwired: 1 in]
        n146 = Index Array(array=w365) -> (element=w362:dbl)  [unwired: 1 in]
        n147 = Index Array(array=w364) -> (element=w363:dbl)  [unwired: 1 in]
        n148 = Get Date/Time String(want seconds? (F)=TRUE) -> (date string=w388:string, time string=w387:string)  [unwired: 2 in]
        n149 = Get Date/Time String(want seconds? (F)=TRUE) -> (date string=w384:string, time string=w385:string)  [unwired: 2 in]
        n150 = Get Date/Time String(want seconds? (F)=TRUE) -> (date string=w371:string, time string=w370:string)  [unwired: 2 in]
        n151 = Format Into String(format string="%s\\s%s\\s%f\\n", w388, w387, w361) -> (resulting string=w398:string)  [unwired: 2 in, 1 out]
        n152 = Format Into String(format string="%s\\s%s\\s%f\\n", w384, w385, w362) -> (resulting string=w380:string)  [unwired: 2 in, 1 out]
        n153 = Format Into String(format string="%s\\s%s\\s%f\\n", w371, w370, w363) -> (resulting string=w375:string)  [unwired: 2 in, 1 out]
        n154 = feedback #1() -> (w395:string[])  [unwired: 1 in]
        n155 = Build Array (concatenate)(w398, w395) -> (w394:string[])
        n156 = feedback-in #1(w394) -> ()
        n157 = feedback #2() -> (w382:string[])  [unwired: 1 in]
        n158 = Build Array (concatenate)(w380, w382) -> (w383:string[])
        n159 = feedback-in #2(w383) -> ()
        n160 = feedback #3() -> (w373:string[])  [unwired: 1 in]
        n161 = Build Array (concatenate)(w375, w373) -> (w372:string[])
        n162 = feedback-in #3(w372) -> ()
        n163 = Concatenate Strings(w394) -> (w386:string)
        n164 = Concatenate Strings(w383) -> (w378:string)
        n165 = Concatenate Strings(w372) -> (w377:string)
      }
      frame Error {
      }
    }
    "MtM X-Axis Output Voltage" <- w355
    "MtM Y-Axis Output Voltage" <- w354
    "MtM Z-Axis Output Voltage" <- w353
    n166 = shared-variable "NI-PXIe-8880\\Shared Variable Library.lvlib\\Data Record Work Rate"("Data History Work Rate (ms)") -> ()  [unwired: 1 in, 1 out]
    n167 = Wait (ms)(milliseconds to wait="Data History Work Rate (ms)") -> ()  [unwired: 1 out]
    n168 = call <extravilib>:"Read.vi"("channel"=w358) -> ("element"=w357:bool)  [unwired: 1 in, 1 out]
  }
  n169 = call-poly <vilib>:"DAQmx Write.vi"("task/channels in"=w34, "data"=0.0 ("Waveform"), "error in"=w33) -> ("task out"=w36:refnum<k21>, "error out"=w35:errorcluster)  [unwired: 10 in, 1 out]
  n170 = call <vilib>:"DAQmx Stop Task.vi"("task/channels in"=w36, "error in"=w35) -> ("task out"=w38:refnum<k21>, "error out"=w37:errorcluster)  [unwired: 12 in]
  n171 = call <vilib>:"DAQmx Clear Task.vi"("task in"=w38, "error in"=w37) -> ()  [unwired: 13 in, 1 out]
  n172 = call <vilib>:"DAQmx Stop Task.vi"("task/channels in"=w87, "error in"=w86) -> ("task out"=w84:refnum<k21>, "error out"=w85:errorcluster)  [unwired: 12 in]
  n173 = call <vilib>:"DAQmx Clear Task.vi"("task in"=w84, "error in"=w85) -> ()  [unwired: 13 in, 1 out]
  n174 = disable-structure shown="Disabled" {
    disable-tunnel: w28 -> [w399 _]
    frame Disabled {
      w411 = 10390 items=["Sample Clock"=10388, "Burst Handshake"=12548, "Handshake"=10389, "Implicit"=10451, "On Demand"=10390, "Change Detection"=12504, "Pipelined Sample Clock"=14668] ("SampTimingType")
      w416 = -1 items=["Default"=-1, "RSE"=10083, "Differential"=10106, "Pseudodifferential"=12529] ("output terminal configuration")
      n175 = call-poly <vilib>:"DAQmx Create Virtual Channel.vi"("output terminal configuration"=w416, "physical channels"=tag "PXIe-6739/ao63:61") -> ("task out"=w413:refnum<k21>, "error out"=w412:errorcluster)  [unwired: 12 in]
      n176 = property class="DAQmx Timing"(reference=w413, error in=w412, "SampTimingType"=w411, "SimultaneousAOEnable"=TRUE) -> (reference out=w415:refnum<k21>, error out=w414:errorcluster)
      n177 = call <vilib>:"DAQmx Start Task.vi"("task/channels in"=w415, "error in"=w414) -> ("task out"=w408:refnum<k21>, "error out"=w407:errorcluster)  [unwired: 12 in]
      n178 = while {
        tunnel: w408 -> [w427]
        tunnel: w407 -> [w426]
        tunnel: [w425] -> w401
        tunnel: [w424] -> w400
        tunnel: w399 -> [w423]
        stop <- w422 stop-if-true
        n179 = case shown="True" "Simulation On/Off" {
          tunnel: w427 -> [w429 w448]
          tunnel: w426 -> [w428 w447]
          tunnel: [w431 w446] -> w425
          tunnel: [w430 w445] -> w424
          tunnel: "MtM Z-Axis Input Voltage" -> [_ w444]
          tunnel: "MtM Y-Axis Input Voltage" -> [_ w443]
          tunnel: "MtM X-Axis Input Voltage" -> [_ w442]
          frame False {
            n180 = call-poly <vilib>:"DAQmx Write.vi"("task/channels in"=w429, "data"=dbl[] [0.0, 0.0, 0.0], "error in"=w428) -> ("task out"=w431:refnum<k21>, "error out"=w430:errorcluster)  [unwired: 10 in, 1 out]
            n181 = property on="MtM Y-Axis Input Voltage" class="DigNum (strict)"("DisabledEnum"=T2."Disabled and Grayed Out" ("Disabled"), "Value"=0.0 ("MtM X-Axis Input Voltage")) -> ()  [unwired: 2 in, 2 out]
            n182 = property on="MtM X-Axis Input Voltage" class="DigNum (strict)"("DisabledEnum"=T2."Disabled and Grayed Out" ("Disabled"), "Value"=0.0 ("MtM X-Axis Input Voltage")) -> ()  [unwired: 2 in, 2 out]
            n183 = property on="MtM Z-Axis Input Voltage" class="DigNum (strict)"("DisabledEnum"=T2."Disabled and Grayed Out" ("Disabled"), "Value"=0.0 ("MtM X-Axis Input Voltage")) -> ()  [unwired: 2 in, 2 out]
          }
          frame True {
            n184 = Build Array(w442, w443, w444) -> (w449:dbl[])  [unwired: 1 in]
            n185 = property on="MtM Y-Axis Input Voltage" class="DigNum (strict)"("DisabledEnum"=T2."Enabled" ("Disabled")) -> ()  [unwired: 2 in, 2 out]
            n186 = property on="MtM Z-Axis Input Voltage" class="DigNum (strict)"("DisabledEnum"=T2."Enabled" ("Disabled")) -> ()  [unwired: 2 in, 2 out]
            n187 = property on="MtM X-Axis Input Voltage" class="DigNum (strict)"("DisabledEnum"=T2."Enabled" ("Disabled")) -> ()  [unwired: 2 in, 2 out]
            n188 = call-poly <vilib>:"DAQmx Write.vi"("task/channels in"=w448, "data"=w449, "error in"=w447) -> ("task out"=w446:refnum<k21>, "error out"=w445:errorcluster)  [unwired: 10 in, 1 out]
          }
        }
        n189 = Wait (ms)(milliseconds to wait=u32 100) -> ()  [unwired: 1 out]
        n190 = call <extravilib>:"Read.vi"("channel"=w423) -> ("element"=w422:bool)  [unwired: 1 in, 1 out]
      }
      n191 = call-poly <vilib>:"DAQmx Write.vi"("task/channels in"=w401, "data"=dbl[] [0.0, 0.0, 0.0], "error in"=w400) -> ("task out"=w404:refnum<k21>, "error out"=w403:errorcluster)  [unwired: 10 in, 1 out]
      n192 = call <vilib>:"DAQmx Stop Task.vi"("task/channels in"=w404, "error in"=w403) -> ("task out"=w406:refnum<k21>, "error out"=w405:errorcluster)  [unwired: 12 in]
      n193 = call <vilib>:"DAQmx Clear Task.vi"("task in"=w406, "error in"=w405) -> ()  [unwired: 13 in, 1 out]
    }
    frame Enabled {
    }
  }
  n194 = Get Date/Time In Seconds() -> (seconds since 1Jan1904=w26:timestamp)
  n195 = TCP Close Connection(connection ID=w71, error in (no error)=w70) -> ()  [unwired: 1 in, 2 out]
  n196 = Format Date/Time String(time format string (%c)="%H.%M.%S", seconds (now)=w26, UTC format=FALSE) -> (date/time string=w18:string)
  n197 = Get Date/Time In Seconds() -> (seconds since 1Jan1904=w23:timestamp)
  n198 = Format Date/Time String(time format string (%c)="%d.%m.%Y", seconds (now)=w23, UTC format=FALSE) -> (date/time string=w19:string)
  n199 = Strip Path(path=path "/home/lvuser/natinst/bin/TestFile/Magnetometer Test/25.07.2024_Test1.xlsx") -> (stripped path=w69:path)  [unwired: 1 out]
  n200 = Format Into String(format string="%s%s%s%s%s%s", w19, w16, w18, w16, "Magnetometer Test" ("input 1"), ".csv" ("input 5")) -> (resulting string=w1:string)  [unwired: 2 in, 1 out]
  n201 = Build Path(base path=w69, name or relative path=w1) -> (appended path=w3:path)
  n202 = call-poly <vilib>:"Write Delimited Spreadsheet.vi"("file path (dialog if empty)"=w3, "1D data"=string[] ["Date", "Time", "X-Axis (V)", "Y-Axis (V)", "Z-Axis (V)", "Temperature", "Output Voltage 1", "Output Current 1", "Output Voltage 2", "Output Current 2", "Magnetic Field", "Output On/Off"]) -> ("new file path (Not A Path if cancelled)"=w68:path, "error out"=w67:errorcluster)  [unwired: 12 in]
  n203 = while {
    tunnel: w68 -> [w474]
    tunnel: w67 -> [w473]
    tunnel: w28 -> [w471]
    stop <- w472 stop-if-true
    n204 = call <extravilib>:"Read.vi"("channel"=w471) -> ("element"=w472:bool)  [unwired: 1 in, 1 out]
    n205 = local read "Output 1 Measured Voltage"() -> (w465:string)
    n206 = local read "Output 2 Measured Current"() -> (w460:string)
    n207 = local read "Output 2 Measured Voltage"() -> (w459:string)
    n208 = local read "Output 2 Measured Current"() -> (w458:string)
    n209 = local read "Temperature (Celsius)"() -> (w450:dbl)
    n210 = local read "Magnetic Field"() -> (w452:dbl)
    n211 = local read "Output On/Off"() -> (w457:bool)
    n212 = Get Date/Time In Seconds() -> (seconds since 1Jan1904=w463:timestamp)
    n213 = shared-variable "NI-PXIe-8880\\Shared Variable Library.lvlib\\X-Axis"() -> (w469:string)  [unwired: 1 in, 1 out]
    n214 = shared-variable "NI-PXIe-8880\\Shared Variable Library.lvlib\\Z-Axis"() -> (w467:string)  [unwired: 1 in, 1 out]
    n215 = shared-variable "NI-PXIe-8880\\Shared Variable Library.lvlib\\Y-Axis"() -> (w468:string)  [unwired: 1 in, 1 out]
    n216 = Get Date/Time String(seconds (now)=w463, want seconds? (F)=TRUE) -> (date string=w462:string, time string=w461:string)  [unwired: 1 in]
    n217 = Boolean To (0,1)(Boolean=w457) -> (0, 1=w456:i16)
    n218 = Number To Fractional String(number=w450) -> (F-format string=w453:string)  [unwired: 3 in]
    n219 = Number To Fractional String(number=w452) -> (F-format string=w454:string)  [unwired: 3 in]
    n220 = Number To Decimal String(number=w456) -> (decimal integer string=w455:string)  [unwired: 1 in]
    n221 = Build Array(w462, w461, w469, w468, w467, w453, w465, w460, w459, w458, w454, w455) -> (w466:string[])
    n222 = call-poly <vilib>:"Write Delimited Spreadsheet.vi"("file path (dialog if empty)"=w474, "1D data"=w466, "append to file? (new file:F)"=TRUE, "error in (no error)"=w473) -> ()  [unwired: 10 in, 2 out]
    n223 = Wait (ms)(milliseconds to wait="Data Record Work Rate (ms)") -> ()  [unwired: 1 out]
  }
  n224 = disable-structure shown="Disabled" {
    disable-tunnel: w28 -> [w476 _]
    frame Disabled {
      n225 = TCP Open Connection(address="10.0.194.41", remote port or service name=u16 6444) -> (connection ID=w481:refnum<k5>, error out=w479:errorcluster)  [unwired: 3 in]
      n226 = while {
        tunnel: w481 -> [w494]
        tunnel: [w493] -> w480
        tunnel: w479 -> [w492]
        tunnel: [w491] -> w478
        tunnel: w476 -> [w484]
        stop <- w485 stop-if-true
        n227 = call <extravilib>:"Read.vi"("channel"=w484) -> ("element"=w485:bool)  [unwired: 1 in, 1 out]
        n228 = shared-variable "NI-PXIe-8880\\Shared Variable Library.lvlib\\X-Axis"() -> (w488:string)  [unwired: 1 in, 1 out]
        n229 = shared-variable "NI-PXIe-8880\\Shared Variable Library.lvlib\\Z-Axis"() -> (w486:string)  [unwired: 1 in, 1 out]
        n230 = shared-variable "NI-PXIe-8880\\Shared Variable Library.lvlib\\Y-Axis"() -> (w487:string)  [unwired: 1 in, 1 out]
        n231 = local read item#-1() -> (w489)
        n232 = Format Into String(format string="%s,%s,%s,%f", w488, w487, w486, w489) -> (resulting string=w490:string)  [unwired: 2 in, 1 out]
        n233 = TCP Write(connection ID=w494, data in=w490, error in (no error)=w492, 9:1 ("timeout ms (25000)")) -> (connection ID out=w493:refnum<k5>, error out=w491:errorcluster)  [unwired: 1 out]
      }
      n234 = TCP Close Connection(connection ID=w480, error in (no error)=w478) -> ()  [unwired: 1 in, 2 out]
    }
    frame Enabled {
    }
  }
  n235 = flat-sequence {
    frame #0 {
      n236 = Current VI's Path() -> (path=w496:path)
      n237 = Open VI Reference(vi path=w496) -> (vi reference=w495:refnum<vi>)  [unwired: 5 in, 1 out]
      n238 = invoke class="VI" method="Default Vals.Reinit All"(reference=w495) -> ()  [unwired: 2 in, 3 out]
    }
  }
